vi "String-NumberToBool.vi"(9 "Numeric":dbl, 10 "String":string) -> (2 "Boolean":bool)   [LabVIEW 2018]
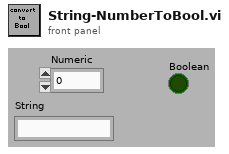
[diagram p1: front panel]
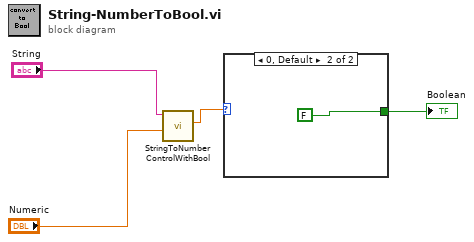
[diagram p0: block diagram]
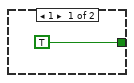
[diagram p2: hidden frame]
diagram:
  n1 = call "StringToNumberControlWithBool.vi"("Numeric In"="Numeric", "String In"="String") -> ("Number Out"=w3:dbl)  [unwired: 6 in, 1 out]
  n2 = case shown="0, Default" w3 {
    tunnel: [TRUE FALSE] -> w4
    frame 1 {
    }
    frame 0, Default {
    }
  }
  "Boolean" <- w4
